vi "Emergency Send To Specific Target.vi"(8 "error in (no error)":errorcluster, 9 "Mail Strategy In":refnum<class "Mail Strategy.lvclass">, 10 "Message In":refnum<class "Message.lvclass">, 11 "Messenger in":refnum<class "Tree-ArrayLocation Queue Messenger.lvclass">) -> (0 "error out":errorcluster, 3 "Messenger out":refnum<class "Tree-ArrayLocation Queue Messenger.lvclass">)   [LabVIEW 2019, in "Tree-ArrayLocation Queue Messenger.lvclass"]
uses:
  Tree-ArrayLocation Queue Messenger.lvclass
  C:/Users/iio/Desktop/NTHU Brain Center/General Purpose/Classes/Ancestor/Messenger/Messenger Composite/Messenger Composite.lvclass
  Ancestor Class/Message/Message.lvclass
  Ancestor Class/Messenger/Mail Strategy/Mail Strategy.lvclass
  Array Location Mailman/Array Location Mailman.lvclass
  C:/Users/iio/Desktop/NTHU Brain Center/General Purpose/Classes/Ancestor/Messenger/Mail Strategy/Mail Strategy.lvclass
  Array Location Mailman/Array Location Mailman.lvclass/Array Location Mailman.ctl
  Ancestor Class/Messenger/Messenger Composite/Messenger Composite.lvclass/Messenger Composite.ctl
  Tree-ArrayLocation Queue Messenger.lvclass/Tree-ArrayLocation Queue Messenger.ctl
  Array Location Mailman/Public Data/Write Location.vi
  Ancestor Class/Messenger/Messenger Composite/Public Data/Read Nodes.vi
  Array Location Mailman/Public Data/Read Location.vi
  Ancestor Class/Messenger/Messenger/Messenger.lvclass
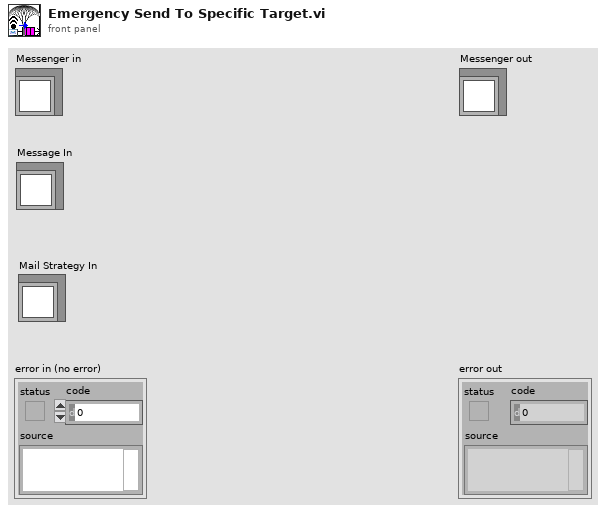
[diagram p1: front panel]
types:
  T1 = typedef "Message Queue.ctl" = refnum<queue>
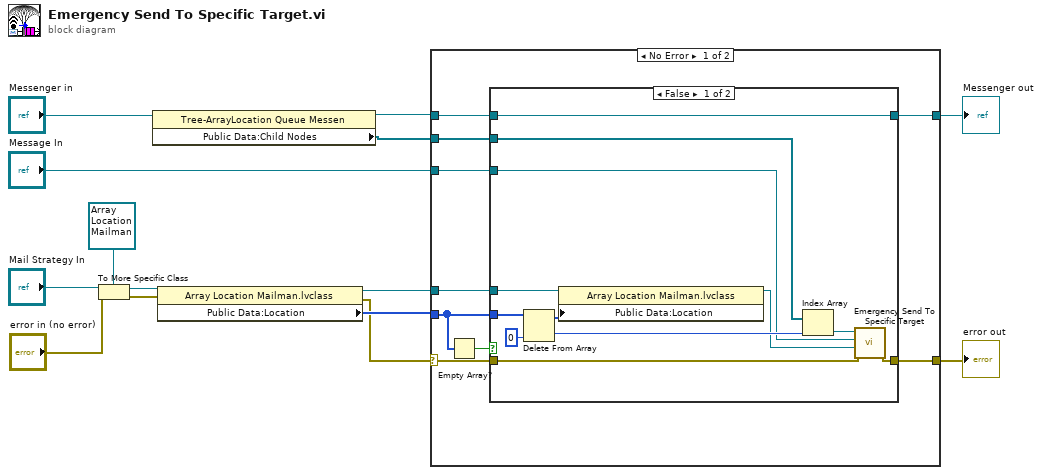
[diagram p0: block diagram]
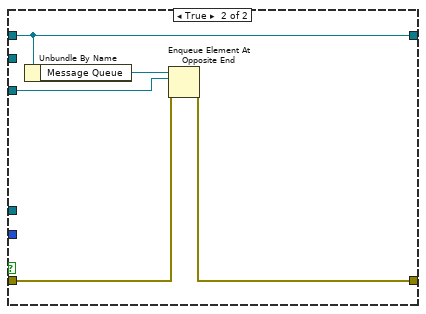
[diagram p2: hidden frame]
diagram:
  n1 = To More Specific Class(target class=refnum<class "Array Location Mailman.lvclass"> refnum ("Array Location Mailman.lvclass"), reference="Mail Strategy In", error in="error in (no error)") -> (specific class reference=w7:refnum<class "Array Location Mailman.lvclass">, error out=w8:errorcluster)
  n2 = property class="Tree-ArrayLocation Queue Messen"(reference="Messenger in") -> (reference out=w2:refnum<class "Tree-ArrayLocation Queue Messenger.lvclass">, "Public Data:Child Nodes"=w1:refnum<class "Messenger.lvclass">[])  [unwired: 1 in, 1 out]
  n3 = property class="Array Location Mailman.lvclass"(reference=w7, error in=w8) -> (reference out=w4:refnum<class "Array Location Mailman.lvclass">, error out=w5:errorcluster, "Public Data:Location"=w6:i32[])
  n4 = case shown="No Error" w5 {
    selector: w5 -> [w18 w41]
    tunnel: w2 -> [w22 w42]
    tunnel: [w20 w42] -> w14
    tunnel: [w17 w41] -> w12
    tunnel: w6 -> [w19 _]
    tunnel: "Message In" -> [w21 _]
    tunnel: w4 -> [w15 _]
    tunnel: w1 -> [w16 _]
    frame No Error {
      n5 = Empty Array?(array=w19) -> (empty?=w23:bool)
      n6 = case shown="False" w23 {
        tunnel: w22 -> [w35 w40]
        tunnel: w21 -> [w30 w38]
        tunnel: [w35 w40] -> w20
        tunnel: w19 -> [w34 _]
        tunnel: w18 -> [w29 w37]
        tunnel: [w28 w36] -> w17
        tunnel: w16 -> [w27 _]
        tunnel: w15 -> [w25 _]
        frame False {
          n7 = Delete From Array(array=w34, index=0) -> (deleted portion=w32:i32, array with subset deleted=w26:i32[])  [unwired: 1 in]
          n8 = property class="Array Location Mailman.lvclass"(reference=w25, "Public Data:Location"=w26) -> (reference out=w24:refnum<class "Array Location Mailman.lvclass">)  [unwired: 1 in, 1 out]
          n9 = Index Array(array=w27, index=w32) -> (element=w31:refnum<class "Messenger.lvclass">)
          n10 = call-dynamic "Emergency Send To Specific Target.vi"("error in (no error)"=w29, "Mail Strategy In"=w24, "Message In"=w30, "Messenger in"=w31) -> ("error out"=w28:errorcluster)  [unwired: 6 in, 1 out]
        }
        frame True {
          n11 = Unbundle By Name(w40) -> ("Message Queue"=w39:T1)
          n12 = Enqueue Element At Opposite End(queue=w39, element=w38, error in (no error)=w37) -> (error out=w36:errorcluster)  [unwired: 1 in, 2 out]
        }
      }
    }
    frame Error {
    }
  }
  "error out" <- w12
  "Messenger out" <- w14
